vi "Bridge.vi"   [LabVIEW 2013]
uses:
  Robot Global Data.vi
types:
  T1 = cluster{"Activate Elevator":bool, "Shoot":bool, "Bridge Direction":bool, "Low Speed":bool, "Med Speed":bool, "High Speed":bool, "Loader Down":bool, "Activate Bridge":bool, "Limit Shooter":bool, "Elevator Down":bool, "Reverse":bool, "Vision Processing":bool}
  T2 = typedef "WPI_DigitalInputDevRef.ctl" = cluster{"DevStatus":errorcluster, "DIO Channel":T3, "Digital Module":T4}
  T3 = typedef "FPGA_DIOChannel.ctl" = enum8{"DIO 1", "DIO 2", "DIO 3", "DIO 4", "DIO 5", "DIO 6", "DIO 7", "DIO 8", "DIO 9", "DIO 10", "DIO 11", "DIO 12", "DIO 13", "DIO 14", "Invalid"}
  T4 = typedef "FPGA_TypedefDigitalModule.ctl" = enum16{"Digital Module 1", "Digital Module 2"}
  T5 = typedef "WPI_MotorControlDeviceRef.ctl" = cluster{"DeviceStatus":errorcluster, "Type":enum16{"PWM", "CAN"}, "PWM":cluster{"Digital Module":T4, "PWM Channel":T6, "DeadBand":T7}, "CAN":cluster{"Device Number":u8, "Control Mode":T8, "Semaphore":T9, "Max Vout":dbl}, "Invert":bool, "TransformRef":T10, "InvTransformRef":T10}
  T6 = typedef "FPGA_DIOPWMChannel.ctl" = enum8{"PWM 1", "PWM 2", "PWM 3", "PWM 4", "PWM 5", "PWM 6", "PWM 7", "PWM 8", "PWM 9", "PWM 10", "Invalid"}
  T7 = typedef "WPI_PWMDeadband.ctl" = cluster{"Name":string, "maxPositivePwm":i32, "minPositivePwm":i32, "centerPwm":i32, "maxNegativePwm":i32, "minNegativePwm":i32, "angularRange":u16}
  T8 = typedef "WPI_CANJaguar_ControlMode.ctl" = enum8{"Percent VBus", "Current", "Speed", "Position", "Voltage"}
  T9 = typedef "Semaphore RefNum" = refnum<k1>
  T10 = typedef "WPI_PWMTransform_ConPane.ctl" = refnum<vi>
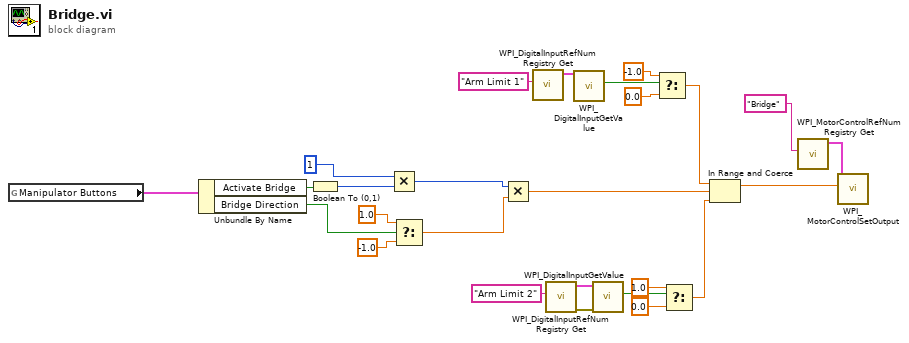
[diagram p0: block diagram]
diagram:
  n1 = global read "Robot Global Data.vi" "Manipulator Buttons"() -> (w26:T1)
  n2 = Unbundle By Name(w26) -> ("Activate Bridge"=w12:bool, "Bridge Direction"=w7:bool)
  n3 = Boolean To (0,1)(Boolean=w12) -> (0, 1=w11:i16)
  n4 = Multiply(x=1, y=w11) -> (x*y=w4:i32)
  n5 = Select(t=1.0, s=w7, f=-1.0) -> (s? t:f=w3:dbl)
  n6 = Multiply(x=w4, y=w3) -> (x*y=w2:dbl)
  n7 = call <vilib>:"WPI_DigitalInputRefNum Registry Get.vi"("refnum name"="Arm Limit 1") -> ("DigitalInputDevRef"=w16:T2)  [unwired: 9 in, 1 out]
  n8 = call <vilib>:"WPI_DigitalInputRefNum Registry Get.vi"("refnum name"="Arm Limit 2") -> ("error out"=w22:errorcluster, "DigitalInputDevRef"=w21:T2)  [unwired: 9 in]
  n9 = call <vilib>:"WPI_DigitalInputGetValue.vi"("DigitalInputDevRef"=w16) -> ("Value"=w8:bool)  [unwired: 8 in, 2 out]
  n10 = call <vilib>:"WPI_DigitalInputGetValue.vi"("error in (no error)"=w22, "DigitalInputDevRef"=w21) -> ("Value"=w20:bool)  [unwired: 7 in, 2 out]
  n11 = Select(t=-1.0, s=w8, f=0.0) -> (s? t:f=w15:dbl)
  n12 = Select(t=1.0, s=w20, f=0.0) -> (s? t:f=w17:dbl)
  n13 = In Range and Coerce(upper limit=w15, x=w2, lower limit=w17) -> (coerced(x)=w14:dbl)  [unwired: 1 out]
  n14 = call <vilib>:"WPI_MotorControlRefNum Registry Get.vi"("refnum name"="Bridge") -> ("MotorControlDevRef"=w13:T5)  [unwired: 9 in, 1 out]
  n15 = call <vilib>:"WPI_MotorControlSetOutput.vi"("Output"=w14, "MotorControlDevRef"=w13) -> ()  [unwired: 7 in, 3 out]
